vi "Read Report Queue.vi"(8 "error in (no error)":errorcluster, 11 "Engine in":refnum<class "Engine.lvclass">) -> (0 "error out":errorcluster, 2 "Report Queue":refnum<class "QDMH.lvclass">, 3 "Engine out":refnum<class "Engine.lvclass">)   [LabVIEW 2023, in "Engine.lvlib" / "Engine.lvclass"]
uses:
  Project/Engine.lvclass
  builds/Tools/QDMH.lvlibp/QDMH.lvclass
  Project/Engine.lvclass/Engine.ctl
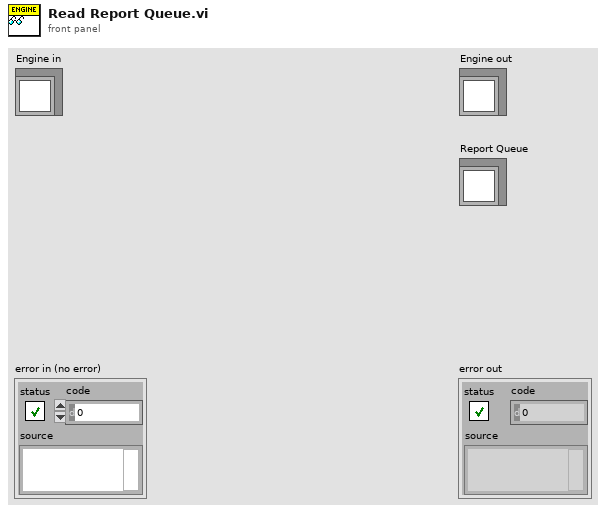
[diagram p1: front panel]
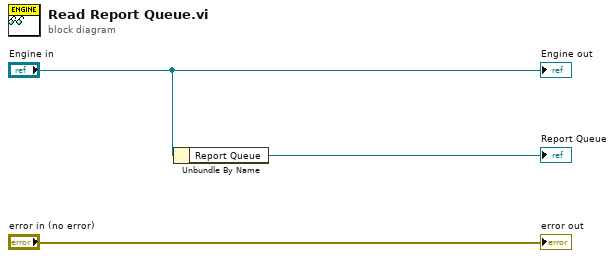
[diagram p0: block diagram]
diagram:
  n1 = Unbundle By Name("Engine in") -> ("Report Queue"=→"Report Queue":refnum<class "QDMH.lvclass">)
  "error out" <- "error in (no error)"
  "Engine out" <- "Engine in"
